vi "MicroSlide-Execute.vi"(0 "VISA resource name":refnum<visa-resource-name>="COM15", 2 "Commande":u16(ring) items=["Initialisation", "Mise dans le faisceau", "Retirer du faisceau"], 11 "Error IN":errorcluster) -> (4 "VRN OUT":refnum<visa-resource-name>, 8 "Erreur":bool, 13 "Received Buffer":string, 15 "Error OUT":errorcluster)   [LabVIEW 2019]
panel:
  in  "Timeout(ms)":dbl=60000.0
  out "Done!":bool
  out "Active":bool
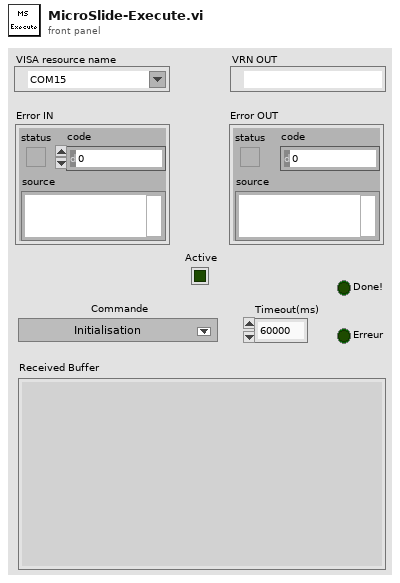
[diagram p1: front panel]
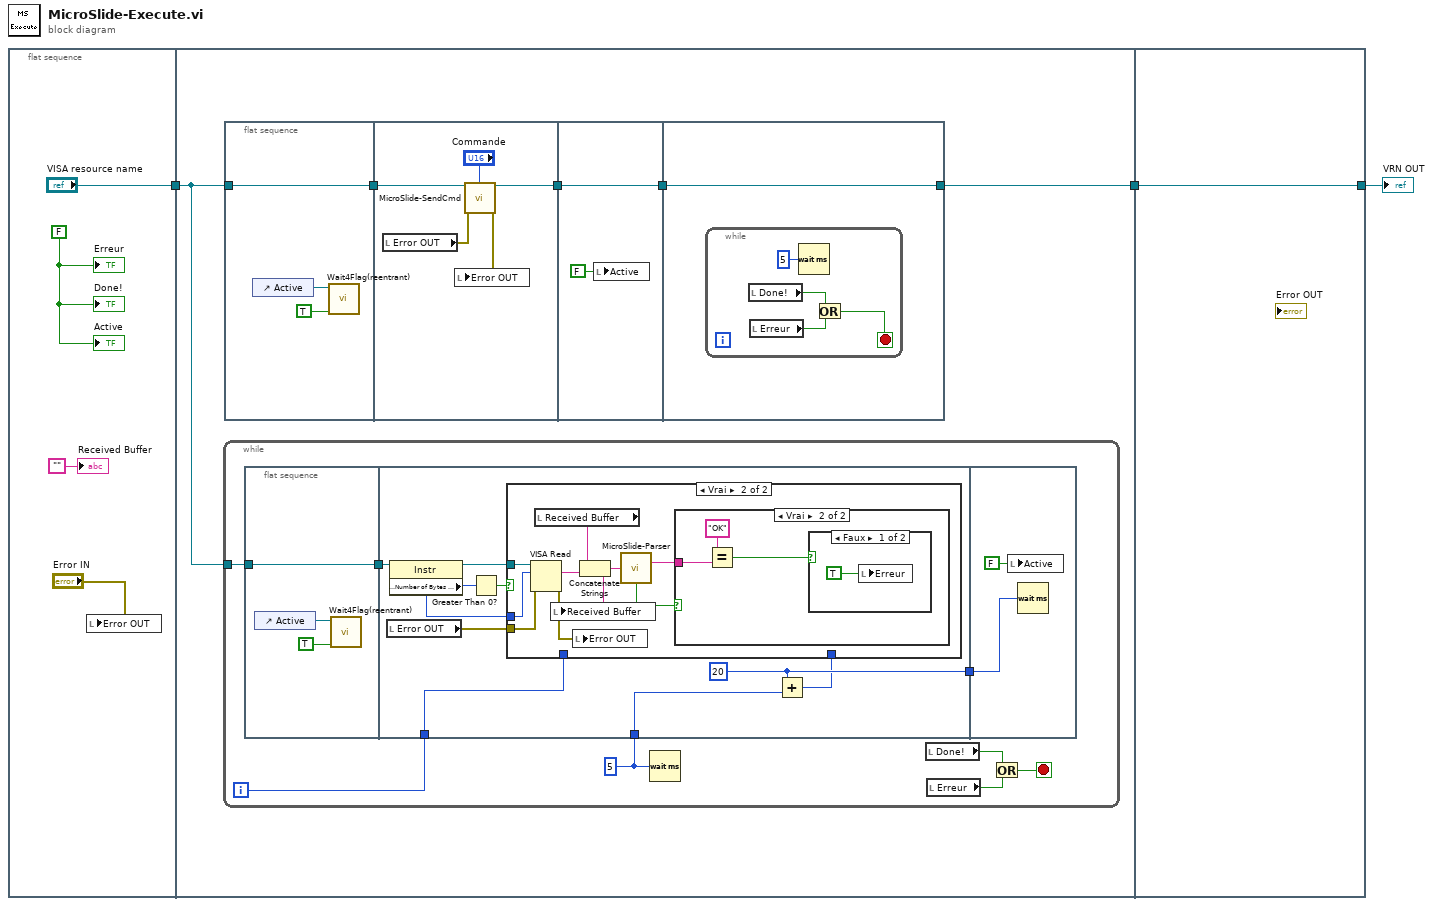
[diagram p0: block diagram]
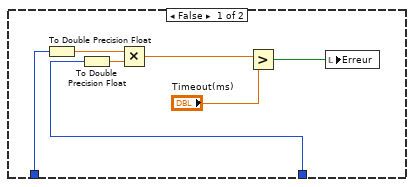
[diagram p2: hidden frame]
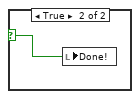
[diagram p4: hidden frame]
diagram:
  n1 = flat-sequence {
    tunnel: ["VISA resource name"] -> w3
    tunnel: w3 -> [w12]
    tunnel: [w11] -> w1
    tunnel: [w71] -> w2
    tunnel: w1 -> [w71]
    frame #0 {
      w5 = FALSE ("Enable Termination\nChar (T)")
      n2 = local write "Error OUT"("Error IN") -> ()
      "Active" <- w5
      "Received Buffer" <- ""
      "Done!" <- w5
      "Erreur" <- w5
    }
    frame #1 {
      n3 = while {
        tunnel: w12 -> [w35]
        i -> [w30]
        stop <- w31 stop-if-true
        w29 = u32 5 ("milliseconds to wait")
        n4 = flat-sequence {
          tunnel: w35 -> [w38]
          tunnel: [w38] -> w34
          tunnel: w34 -> [w47]
          tunnel: w30 -> [w42]
          tunnel: w29 -> [w41]
          tunnel: [w40] -> w28
          tunnel: w28 -> [w69]
          frame #0 {
            n5 = control-ref of="Active"() -> (w36:refnum<vi>)
            n6 = call "Wait4Flag(reentrant).vi"("Raise Flag ?"=TRUE, "Ctl Refnum IN"=w36) -> ()  [unwired: 8 in, 2 out]
          }
          frame #1 {
            w40 = u32 20 ("milliseconds to wait")
            n7 = local read "Error OUT"() -> (w43:errorcluster)
            n8 = property class="Instr"(reference=w47) -> (reference out=w45:refnum<visa-resource-name>, "Serial Settings:Number of Bytes at Serial Port"=w44:u32)  [unwired: 1 in, 1 out]
            n9 = Greater Than 0?(x=w44) -> (x > 0?=w46:bool)
            n10 = Add(x=w40, y=w41) -> (x+y=w39:u32)
            n11 = case shown="Vrai" w46 {
              tunnel: w45 -> [_ w63]
              tunnel: w44 -> [_ w62]
              tunnel: w43 -> [_ w57]
              tunnel: w42 -> [w52 _]
              tunnel: w39 -> [w51 _]
              frame False {
                n12 = To Double Precision Float(number=w52) -> (double precision float=w53:dbl)
                n13 = To Double Precision Float(number=w51) -> (double precision float=w54:dbl)
                n14 = Multiply(x=w53, y=w54) -> (x*y=w50:dbl)
                n15 = Greater?(x=w50, y="Timeout(ms)") -> (0:w48:bool)
                n16 = local write "Erreur"(w48) -> ()
              }
              frame True {
                n17 = VISA Read(VISA resource name=w63, byte count=w62, error in (no error)=w57) -> (read buffer=w59:string, error out=w56:errorcluster)  [unwired: 2 out]
                n18 = local read "Received Buffer"() -> (w60:string)
                n19 = local write "Error OUT"(w56) -> ()
                n20 = Concatenate Strings(w60, w59) -> (w55:string)
                n21 = local write "Received Buffer"(w55) -> ()
                n22 = call "MicroSlide-Parser.vi"("String"=w55) -> ("Answer"=w58:string, "Received"=w61:bool)  [unwired: 12 in, 1 out]
                n23 = case shown="Vrai" w61 {
                  tunnel: w58 -> [_ w66]
                  frame False {
                  }
                  frame True {
                    n24 = Equal?(x="OK", y=w66) -> (x = y?=w64:bool)
                    n25 = case shown="Faux" w64 {
                      selector: w64 -> [_ w68]
                      frame False {
                        n26 = local write "Erreur"(TRUE ("Active")) -> ()
                      }
                      frame True {
                        n27 = local write "Done!"(w68) -> ()
                      }
                    }
                  }
                }
              }
            }
          }
          frame #2 {
            n28 = local write "Active"(FALSE ("Active")) -> ()
            n29 = Wait (ms)(milliseconds to wait=w69) -> ()  [unwired: 1 out]
          }
        }
        n30 = Wait (ms)(milliseconds to wait=w29) -> ()  [unwired: 1 out]
        n31 = local read "Done!"() -> (w33:bool)
        n32 = local read "Erreur"() -> (w32:bool)
        n33 = Or(x=w33, y=w32) -> (x .or. y?=w31:bool)
      }
      n34 = flat-sequence {
        tunnel: w12 -> [w15]
        tunnel: [w15] -> w10
        tunnel: w10 -> [w20]
        tunnel: [w19] -> w9
        tunnel: w9 -> [w21]
        tunnel: [w21] -> w8
        tunnel: [w23] -> w11
        tunnel: w8 -> [w23]
        frame #0 {
          n35 = control-ref of="Active"() -> (w13:refnum<vi>)
          n36 = call "Wait4Flag(reentrant).vi"("Raise Flag ?"=TRUE, "Ctl Refnum IN"=w13) -> ()  [unwired: 8 in, 2 out]
        }
        frame #1 {
          n37 = local read "Error OUT"() -> (w16:errorcluster)
          n38 = call "MicroSlide-SendCmd.vi"("VRN IN"=w20, "Commande"="Commande", "Error IN"=w16) -> ("VRN OUT"=w19:refnum<visa-resource-name>, "Error OUT"=w17:errorcluster)  [unwired: 10 in, 1 out]
          n39 = local write "Error OUT"(w17) -> ()
        }
        frame #2 {
          n40 = local write "Active"(FALSE ("Active")) -> ()
        }
        frame #3 {
          n41 = while {
            stop <- w25 stop-if-true
            n42 = local read "Done!"() -> (w26:bool)
            n43 = local read "Erreur"() -> (w27:bool)
            n44 = Wait (ms)(milliseconds to wait=u32 5) -> ()  [unwired: 1 out]
            n45 = Or(x=w26, y=w27) -> (x .or. y?=w25:bool)
          }
        }
      }
    }
    frame #2 {
    }
  }
  "VRN OUT" <- w2
